vi "LOC subReadWriteVIStringINIKeys(Ring).vi"(4 "Mode":enum16{"Read", "Write"}(ring), 5 "Section":string, 6 "error in (no error)":errorcluster, 8 "ConfigFileRefnum":T1, 9 "ControlRefnum":refnum<vi>) -> (0 "error out":errorcluster)   [LabVIEW 2020, in "Localization_Tools.lvlib"]
uses:
  Localization_Tools.lvlib
  <vilib>/Utility/config.llb/Config Data RefNum.ctl
  <vilib>/Utility/config.llb/NI_LVConfig.lvlib
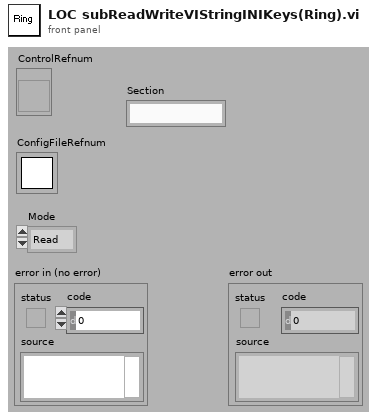
[diagram p1: front panel]
types:
  T1 = typedef "NI_LVConfig.lvlib/Config Data RefNum.ctl" = refnum<k1>
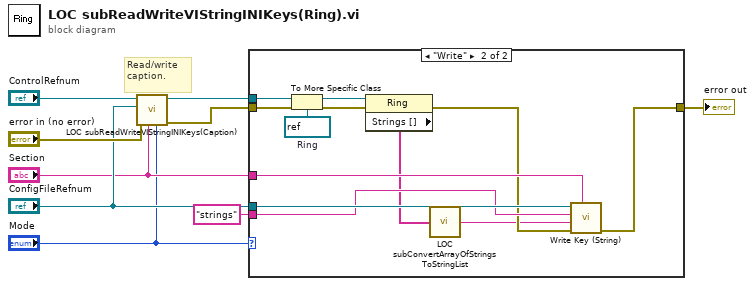
[diagram p0: block diagram]
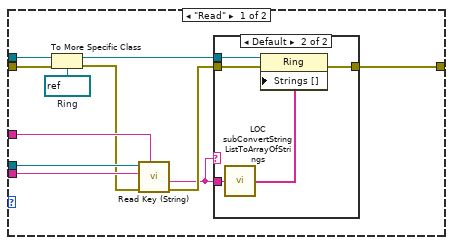
[diagram p2: hidden frame]
diagram:
  # "Read/write\ncaption."
  n1 = call "LOC subReadWriteVIStringINIKeys(Caption).vi"("Mode"="Mode", "Section"="Section", "error in (no error)"="error in (no error)", "ConfigFileRefnum"="ConfigFileRefnum", "ControlRefnum"="ControlRefnum") -> ("error out"=w5:errorcluster, "dup ControlRefnum"=w7:refnum<vi>)  [unwired: 3 in]
  n2 = case shown="\"Write\"" "Mode" {
    tunnel: w7 -> [w16 w37]
    tunnel: w5 -> [w15 w36]
    tunnel: "ConfigFileRefnum" -> [w20 w33]
    tunnel: "Section" -> [w19 w31]
    tunnel: "strings" ("key") -> [w18 w32]
    tunnel: [w11 w29] -> w1
    frame "Read" {
      w17 = refnum<vi> refnum  # Ring
      n3 = To More Specific Class(target class=w17, reference=w16, error in=w15) -> (specific class reference=w13:refnum<vi>, error out=w14:errorcluster)
      n4 = call <vilib>:"Read Key (String).vi"("section"=w19, "error in (no error)"=w14, "key"=w18, "refnum"=w20) -> ("error out"=w12:errorcluster, "value"=w10:string)  [unwired: 4 in, 2 out]
      n5 = case shown="Default" w10 {
        tunnel: w13 -> [_ w26]
        tunnel: w12 -> [w21 w25]
        tunnel: [w21 w24] -> w11
        tunnel: w10 -> [_ w23]
        frame "" {
        }
        frame Default {
          n6 = call "LOC subConvertStringListToArrayOfStrings.vi"("InputString"=w23) -> ("OutputArray"=w22:string[])
          n7 = property class="Ring"(reference=w26, error in=w25, "Strings []"=w22) -> (error out=w24:errorcluster)  [unwired: 1 out]
        }
      }
    }
    frame "Write" {
      w38 = refnum<vi> refnum  # Ring
      n8 = To More Specific Class(target class=w38, reference=w37, error in=w36) -> (specific class reference=w35:refnum<vi>, error out=w34:errorcluster)
      n9 = property class="Ring"(reference=w35, error in=w34) -> (error out=w30:errorcluster, "Strings []"=w28:string[])  [unwired: 1 out]
      n10 = call "LOC subConvertArrayOfStringsToStringList.vi"("InputArray"=w28) -> ("OutputString"=w27:string)
      n11 = call <vilib>:"Write Key (String).vi"("section"=w31, "error in (no error)"=w30, "value"=w27, "key"=w32, "refnum"=w33) -> ("error out"=w29:errorcluster)  [unwired: 4 in, 2 out]
    }
  }
  "error out" <- w1
